vi "Add PWM.vi"(6 "PWM Properties":T1, 8 "error in(no error)":errorcluster, 9 "PWM Name":string, 10 "Read?":bool, 11 "CD Ref in":T2 format="%.0x") -> (0 "error out":errorcluster, 3 "CD Ref out":T2 format="%.0x")   [LabVIEW 2013, in "PWM System Explorer.lvlib"]
uses:
  PWM System Explorer.lvlib
  <vilib>/NI Veristand/Custom Device API/Custom Device Item Ref.ctl
  <vilib>/NI Veristand/Custom Device API/Custom Device Channel.ctl
  <vilib>/NI Veristand/Custom Device API/Custom Device Channel Type.ctl
  Shared/Constants.vi
  <vilib>/NI Veristand/Custom Device API/Custom Device API.lvlib
  Shared/PWM Shared.lvlib
  <vilib>/NI Veristand/Custom Device Tools/Custom Device Utility Library/Custom Device Utility Library.lvlib
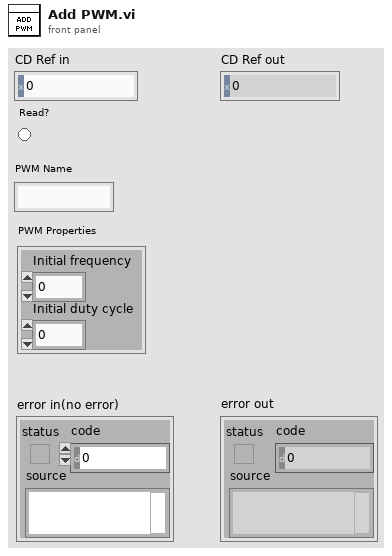
[diagram p1: front panel]
types:
  T1 = cluster{"Initial frequency":dbl, "Initial duty cycle":dbl}
  T2 = typedef "Custom Device API.lvlib/Custom Device Item Ref.ctl" = u64
  T3 = typedef "Custom Device API.lvlib/Custom Device Channel.ctl" = cluster{"Type":T4, "Units":string, "Default Value":dbl, "Faultable":bool, "Scalable":bool}
  T4 = typedef "Custom Device API.lvlib/Custom Device Channel Type.ctl" = enum16{"Input", "Output"}
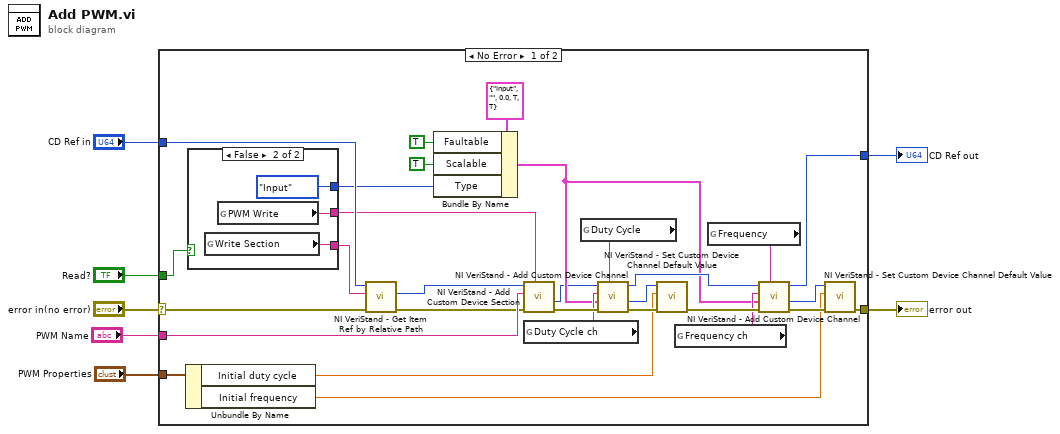
[diagram p0: block diagram]
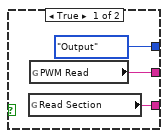
[diagram p2: hidden frame]
diagram:
  n1 = case shown="No Error" "error in(no error)" {
    selector: "error in(no error)" -> [w25 w44]
    tunnel: "Read?" -> [w8 _]
    tunnel: "CD Ref in" -> [w37 w45]
    tunnel: [w27 w45] -> w5
    tunnel: [w26 w44] -> w4
    tunnel: "PWM Name" -> [w17 _]
    tunnel: "PWM Properties" -> [w13 _]
    frame No Error {
      n2 = Unbundle By Name(w13) -> ("Initial duty cycle"=w11:dbl, "Initial frequency"=w12:dbl)
      n3 = case shown="False" w8 {
        tunnel: [w40 w43] -> w36
        tunnel: [w39 w42] -> w35
        tunnel: [Custom_Device_Channel_Type."Output" ("Type") Custom_Device_Channel_Type."Input" ("Type")] -> w21
        frame True {
          n4 = global read "Constants.vi" "Read Section"() -> (w40:string)
          n5 = global read "Constants.vi" "PWM Read"() -> (w39:string)
        }
        frame False {
          n6 = global read "Constants.vi" "Write Section"() -> (w43:string)
          n7 = global read "Constants.vi" "PWM Write"() -> (w42:string)
        }
      }
      n8 = call <vilib>:"NI VeriStand - Get Item Ref by Relative Path.vi"("error in"=w25, "Relative Item Path"=w36, "Section Ref in"=w37) -> ("error out"=w10:errorcluster, "Item Ref"=w9:T2)  [unwired: 5 in, 2 out]
      n9 = Bundle By Name(cluster=T3 {"Type"=enum."Input", "Units"="", "Default Value"=0.0, "Faultable"=TRUE, "Scalable"=TRUE} ("Channel"), "Faultable"=TRUE, "Scalable"=TRUE, "Type"=w21) -> (w18:T3)
      n10 = call <vilib>:"NI VeriStand - Add Custom Device Section.vi"("GUID (Default Section)"=w35, "error in (no error)"=w10, "Section Name"=w17, "Parent Ref in"=w9) -> ("error out"=w33:errorcluster, "Section Ptr"=w16:T2)  [unwired: 4 in, 2 out]
      n11 = global read "Constants.vi" "Duty Cycle ch"() -> (w24:string)
      n12 = global read "Constants.vi" "Duty Cycle"() -> (w14:string)
      n13 = call <vilib>:"NI VeriStand - Add Custom Device Channel.vi"("GUID (Default Channel)"=w14, "error in (no error)"=w33, "Channel"=w18, "Channel Name"=w24, "Parent Ref in"=w16) -> ("error out"=w34:errorcluster, "Channel Ref"=w30:T2, "Parent Ref out"=w29:T2)  [unwired: 3 in, 1 out]
      n14 = call <vilib>:"NI VeriStand - Set Custom Device Channel Default Value.vi"("error in (no error)"=w34, "Default Value"=w11, "Channel Ref in"=w30) -> ("error out"=w31:errorcluster)  [unwired: 7 in, 1 out]
      n15 = global read "Constants.vi" "Frequency ch"() -> (w23:string)
      n16 = global read "Constants.vi" "Frequency"() -> (w15:string)
      n17 = call <vilib>:"NI VeriStand - Add Custom Device Channel.vi"("GUID (Default Channel)"=w15, "error in (no error)"=w31, "Channel"=w18, "Channel Name"=w23, "Parent Ref in"=w29) -> ("error out"=w32:errorcluster, "Channel Ref"=w28:T2, "Parent Ref out"=w27:T2)  [unwired: 3 in, 1 out]
      n18 = call <vilib>:"NI VeriStand - Set Custom Device Channel Default Value.vi"("error in (no error)"=w32, "Default Value"=w12, "Channel Ref in"=w28) -> ("error out"=w26:errorcluster)  [unwired: 7 in, 1 out]
    }
    frame Error {
    }
  }
  "CD Ref out" <- w5
  "error out" <- w4
